vi "Convert from DarkSky API Time.vi"(8 "error in (no error)":errorcluster, 11 "DarkSky Time In":dbl=1501565580.0 format="%#_10g") -> (0 "error out":errorcluster, 3 "Data/Time Out":timestamp=timestamp(3584410380 s since 1904-01-01))   [LabVIEW 2017, in "Dark Sky Weather Data for LabVIEW.lvlib"]
doc: "Use this VI to convert from the time value used by the DarkSky API (UNIX time) to a LabVIEW Date/Time time stamp in UTC format"
uses:
  Dark Sky Weather Data for LabVIEW.lvlib
  <vilib>/Utility/miscctls.llb/LVDateTimeRec.ctl
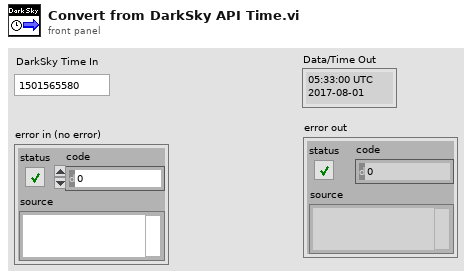
[diagram p1: front panel]
types:
  T1 = typedef "LVDateTimeRec.ctl" = cluster{"fractional second":dbl, "second":i32, "minute":i32, "hour":i32, "day of month":i32, "month":i32, "year":i32, "day of week":i32, "day of year":i32, "DST":i32}
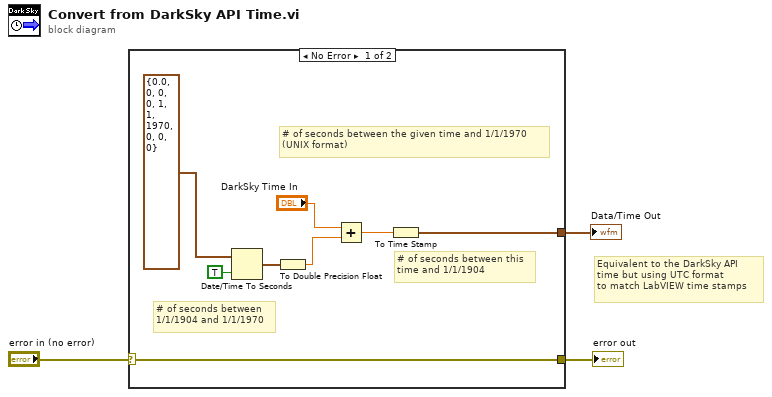
[diagram p0: block diagram]
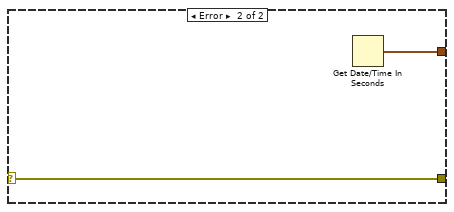
[diagram p2: hidden frame]
diagram:
  # "Equivalent to the DarkSky API\ntime but using UTC format\nto match LabVIEW time stamps"
  n1 = case shown="No Error" "error in (no error)" {
    selector: "error in (no error)" -> [w5 w13]
    tunnel: [w5 w13] -> w2
    tunnel: [w4 w12] -> w1
    frame No Error {
      # "# of seconds between this\ntime and 1/1/1904"
      # "# of seconds between the given time and 1/1/1970\n(UNIX format)"
      # "# of seconds between\n1/1/1904 and 1/1/1970"
      n2 = Date/Time To Seconds(1:TRUE ("is UTC (F)"), 2:T1 {"fractional second"=0.0, "second"=0, "minute"=0, "hour"=0, "day of month"=1, "month"=1, "year"=1970, "day of week"=0, "day of year"=0, "DST"=0} ("date time rec")) -> (0:w9:timestamp)
      n3 = To Double Precision Float(number=w9) -> (double precision float=w7:dbl)
      n4 = Add(x="DarkSky Time In", y=w7) -> (x+y=w6:dbl)
      n5 = To Time Stamp(1:w6) -> (0:w4:timestamp)
    }
    frame Error {
      n6 = Get Date/Time In Seconds() -> (seconds since 1Jan1904=w12:timestamp)
    }
  }
  "Data/Time Out" <- w1
  "error out" <- w2
